vi "DAQ Initialization 4 PID.vi"(8 "error in":errorcluster, 11 "classes in":T2) -> (0 "error out":errorcluster, 3 "classes out":T2)   [LabVIEW 2011]
uses:
  Controls/Class Objects.ctl
  Modules/File/Configuration/Configuration.lvclass
  Modules/Hardware/Power Supply/Power Supply.lvclass
  Modules/Hardware/Mass Flow Controller/Mass Flow Controller.lvclass
  Modules/Hardware/PID/PID.lvclass
  Modules/Hardware/Valve Controller/Valve Controller.lvclass
  Modules/Hardware/Multimeter/Multimeter.lvclass
  Modules/Hardware/Vapour Generator/Vapour Generator.lvclass
  Modules/File/TDMS/TDMS.lvclass
  Controls/DAQ Type.ctl
  Controls/User Interface Action.ctl
  Modules/File/TDMS/File Level.ctl
  Controls/TDMS File Handling.ctl
  Functional Global Data/Device Params Global.ctl
  Functional Global Data/Run Data.ctl
  Functional Global Data/Globals.ctl
  Controls/Display Mode.ctl
  Modules/Hardware/INL PID/INL PID.lvclass
  Modules/Hardware/Baseline Mocon piD-Tech plus/Baseline Mocon piD-Tech plus.lvclass
panel:
  in  "parameter names INL PID":string[](array[string])=["Sampling Frequency", "Integration Time (ms)", "Integration Periods", "Grid Voltage", "Experiment Type", "Notes"]
  in  "Experiment Type":T1
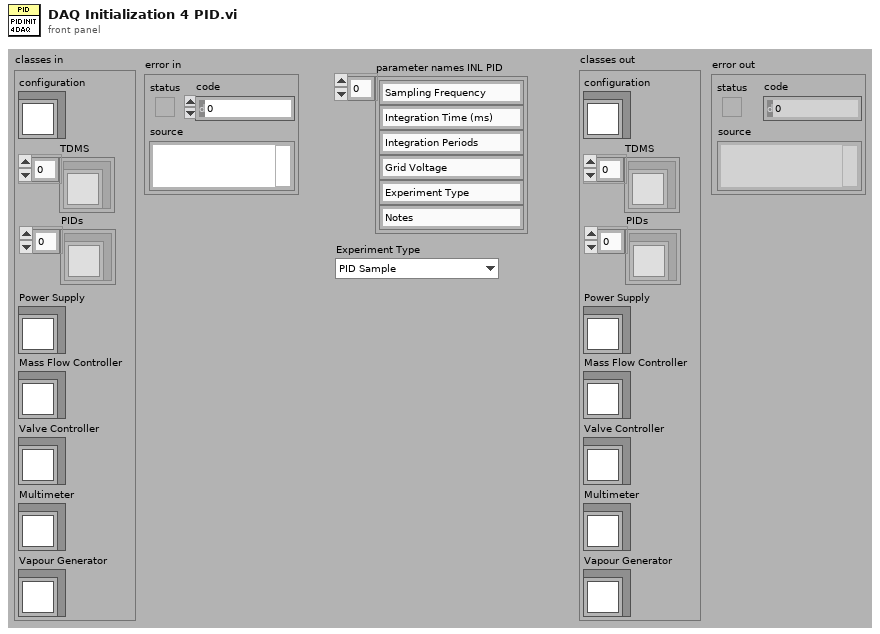
[diagram p1: front panel]
types:
  T1 = typedef "DAQ Type.ctl" = enum16{"PID Sample", "PID with PS Challenge", "PID with MFC Challenge", "Multimeter Sample", "Multimeter with MFC Challenge"}
  T2 = typedef "Class Objects.ctl" = cluster{"configuration":refnum<class "Configuration.lvclass">, "TDMS":refnum<class "TDMS.lvclass">[], "Power Supply":refnum<class "Power Supply.lvclass">, "Mass Flow Controller":refnum<class "Mass Flow Controller.lvclass">, "Valve Controller":refnum<class "Valve Controller.lvclass">, "Multimeter":refnum<class "Multimeter.lvclass">, "Vapour Generator":refnum<class "Vapour Generator.lvclass">, "PIDs":refnum<class "PID.lvclass">[]}
  T3 = typedef "User Interface Action.ctl" = enum16{"Initialize", "Data Acquisition Disable", "Data View Disable", "Sample Set", "Sample Set 2D Data", "Sample Set x0 & dx", "Sample Add", "Sample Set Cursor", "Sample Set Offset & Multiplier", "Sample Set Axis Labels", "Sample Parameters Disabled", "Sample Parameters Update", "Run Update", "Run Set Offset & Multiplier", "Run Set Axis Labels", "Run Set Cursor", "Run Set Disabled", "Run Parameters Update", "Run Parameters Disabled", "Run Number Set", "Run Number Set Range", "Run Number Set Disabled", "Sample Number Set", "Sample Number Set Range", "Notes Set Value", "Update Plot", "Set Plot Parameters", "Update Concentration Plot", "Time Set", "Clear DAQ Display", "Clear Analysis Display", "Status Bar Set", "Progress Bar Set", "Display Mode Set", "Experiment Type Set", "Analysis Plot Average Set", "Stop"}
  T4 = typedef "TDMS.lvclass/File Level.ctl" = enum16{"File", "Group", "Channel"}
  T5 = typedef "TDMS File Handling.ctl" = enum16{"Add TDMS File", "Get Active TDMS File", "Set Active TDMS File", "Set Active TDMS File Index"}
  T6 = typedef "Device Params Global.ctl" = enum16{"Initialize", "Get Device Settings", "Get Device Connections", "Set Device Settings", "Set Device Connections", "Get All Device Properties"}
  T7 = typedef "Run Data.ctl" = enum16{"Initialize", "Add Sample Channel", "Set Run", "Get Number of Runs", "Set Run Params", "Get Spectrum", "Get Run Params", "Get Sample Params", "Get History", "Get Averaged History", "Get Run Param Names", "Set Run Param Names", "Get Sample Param Names", "Set Sample Param Names", "Get MFC Flow Rate Challenge Profile", "Get History Average"}
  T8 = typedef "Globals.ctl" = enum16{"Initialize", "Get DAQ Params", "Get Data Display Params", "Set DAQ Params", "Set Data Display Params"}
  T9 = typedef "Display Mode.ctl" = enum16{"Sample", "Run"}
  T10 = typedef "Device Connections.ctl" = cluster{"Detector":cluster{"Detector Type":T11, "Connection":bool, "B-M PID":T12, "INL PID Connections":T13}, "Power Supply":cluster{"Type":enum16{"Stanford Research PS350", "Keithley 2400"}, "Connection":bool, "VISA resource name":refnum<visa-resource-name>}, "Mass Flow Controller":cluster{"Type":enum16{"Aalborg GFC17"}, "Connection":bool, "Aalborg GFC17":T15}, "Valve Controller":cluster{"Type":T16, "Connection":bool, "SMC - INL":cluster{"VISA resource name":refnum<visa-resource-name>}}, "Multimeter":cluster{"Multimeter Type":T17, "Connection":bool, "VISA resource name":refnum<visa-resource-name>}, "Vapour Generator":cluster{"Type":T18, "Connection":bool, "Owlstone Gen-SYS":T19}}
  T11 = typedef "Detector Type.ctl" = enum16{"INL PID", "Baseline-Mocon piD-TECH plus"}
  T12 = typedef "Baseline Mocon piD-Tech plus.lvclass/Connections.ctl" = cluster{"AI DAQmx channel":tag}
  T13 = typedef "INL PID Connections.ctl" = cluster{"PIDs":u8, "Integrator DAQ Channels 1":T14, "Integrator DAQ Channels 2":T14}
  T14 = typedef "INL PID.lvclass/Integrator DAQmx Channels.ctl" = cluster{"V0":tag, "S1":tag, "S2":tag}
  T15 = typedef "Aalborg GFC17.lvclass/Aalborg GFC17 Connections.ctl" = cluster{"flow rate setpoint channel":tag, "flow rate reading channel":tag, "valve channel":tag}
  T16 = typedef "Valve Type.ctl" = enum16{"SMC - INL"}
  T17 = typedef "Multimeter Type.ctl" = enum16{"Agilent 3458A"}
  T18 = typedef "Vapour Generator Type.ctl" = enum16{"Owlstone GEN-SYS"}
  T19 = typedef "Owlstone GEN-SYS.lvclass/GEN-SYS Connections.ctl" = cluster{"GEN-SYS VISA resource name":refnum<visa-resource-name>, "OVG-4":cluster{"Flow Address":u8, "Temp Address":u8}, "OHG-4":cluster{"Flow Address":u8, "Easydew VISA resource name":refnum<visa-resource-name>}}
  T20 = typedef "Device Settings.ctl" = cluster{"PID":cluster{"B-M PID":T21, "INL PID":T22}, "Power Supply":cluster{"Source Value":dbl, "Source Value Units":T23, "Source Mode":T24, "Limits":T25, "Output":bool}, "Mass Flow Controller":cluster{"MFC Flow Rate":dbl, "MFC Valve Status":T28}, "Valve Controller":cluster{"Valve Assembly":T29}, "Multimeter":cluster{"Agilent 3458A":cluster{"Measurement Configuration":T31, "Measurement Integration":T32}}, "Vapour Generator":cluster{"Owlstone Permeation Tube":T33, "Owlstone GEN-SYS Setpoints":T35}}
  T21 = typedef "Baseline Mocon piD-Tech plus.lvclass/Settings.ctl" = cluster{"Detector Sampling Frequency":dbl}
  T22 = typedef "INL PID.lvclass/Settings.ctl" = cluster{"Sampling Frequency":dbl, "Integration Time":dbl, "Integration Periods":u8, "Grid Voltage":dbl}
  T23 = typedef "Power Supply.lvclass/Source Units.ctl" = enum16{"volts", "millivolts", "microvolts", "amps", "milliamps", "microamps", "nanoamps"}
  T24 = typedef "Power Supply.lvclass/Source Mode.ctl" = enum16{"Volts", "Current"}
  T25 = typedef "Power Supply.lvclass/Protection Limits.ctl" = cluster{"Voltage Limit":dbl, "Voltage Limit Units":T26, "Current Limit":dbl, "Current Limit Units":T27, "Voltage Trip/Cmpl":dbl, "Voltage Trip/Cmpl Units":T26, "Current Trip/Cmpl":dbl, "Current Trip/Cmpl Units":T27}
  T26 = typedef "Power Supply.lvclass/Voltage Units.ctl" = enum16{"volts", "millivolts", "microvolts"}
  T27 = typedef "Power Supply.lvclass/Current Units.ctl" = enum16{"amps", "milliamps", "microamps", "nanoamps"}
  T28 = typedef "Mass Flow Controller.lvclass/Valve Status.ctl" = enum16{"Open", "Closed"}
  T29 = typedef "Valve Controller.lvclass/Valve Assembly.ctl" = cluster{"Valve 1":T30, "Valve 2":T30, "Valve 3":T30, "Valve 4":T30, "Valve 5":T30}
  T30 = typedef "Valve Controller.lvclass/Status.ctl" = u16
  T31 = typedef "Agilent 3458A.lvclass/Measurement Configuration.ctl" = cluster{"Function":enum16{"DC Voltage", "AC Voltage", "AC + DC Voltage", "DC Current", "AC Current", "AC + DC Current", "2-Wire Resistance", "4-Wire Resistance", "Frequency", "Period", "Direct Sampling DC", "Direct Sampling AC", "Sub-Sampling DC", "Sub-Sampling AC"}, " Manual Resolution":enum16{"4.5", "5.5", "6.5", "7.5", "8.5"}, "Frequency Source":enum16{"AC + DC Current", "AC + DC Voltage", "AC Current", "AC Voltage"}, "Auto Range":enum16{"OFF", "ON", "ONCE"}}
  T32 = typedef "Agilent 3458A.lvclass/Measurement Integration.ctl" = cluster{"Power Line Cycles":dbl}
  T33 = typedef "Owlstone GEN-SYS.lvclass/Permeation Tube.ctl" = cluster{"Tube":T34, "Molecular Weight":dbl, "Calibration Temperature\n(Celcius)":i32, "Permeation Rate \n(ng/min)":i32}
  T34 = typedef "Owlstone GEN-SYS.lvclass/Permeation Tube Gas.ctl" = enum16{"Isobutylene 27 Nov 2012", "Ammonia 29 Sep 2012", "DMMP Tube A 3 July 2014", "DMMP Tube B 3 July 2014"}
  T35 = typedef "Owlstone GEN-SYS.lvclass/Gen-Sys Setpoints.ctl" = cluster{"OVG-4":cluster{"Oven Temperature":i32, "Sample Flow Rate":i32, "Split Flow Status":u16, "Split Flow Rate":i32}, "OHG-4":cluster{"Wet Air Flow":i32}}
  T36 = typedef "Data Acquisition Parameters.ctl" = cluster{"Experiment Type":T1, "Experiment Name":string, "Operator Name":string, "Notes":string, "TDMS File Path":path, "Data Acquisition State":bool, "PID Voltage Sweep":T37, "MFC Challenge Profile - Heaviside Step":T38, "MFC Challenge Profile":T39, "MFC Challenge Profile - Staircase":T40}
  T37 = typedef "PID Voltage Seep Settings.ctl" = cluster{"Voltage Step (V)":dbl, "Voltage Range (V)":cluster{u16, u16}, "Time Step (s)":dbl, "Voltage Step Direction":enum16{"High 2 Low", "Low 2 High"}}
  T38 = typedef "MFC Challenge Profile - Heaviside Step.ctl" = cluster{"Valve Open Duration":u16, "MFC Flow Rate":dbl, "Valve Open Repeats":u16, "Valve Open Start":u16}
  T39 = typedef "MFC Challen Profile Type.ctl" = enum16{"Heaviside", "Staircase"}
  T40 = typedef "MFC Challenge Profile - Staircase.ctl" = cluster{"Step Time Duration":u16, "Step Flow Rate":dbl, "Steps":u16, "Valve Open Start":u16, "Recovery":bool, "Repeats":u16}
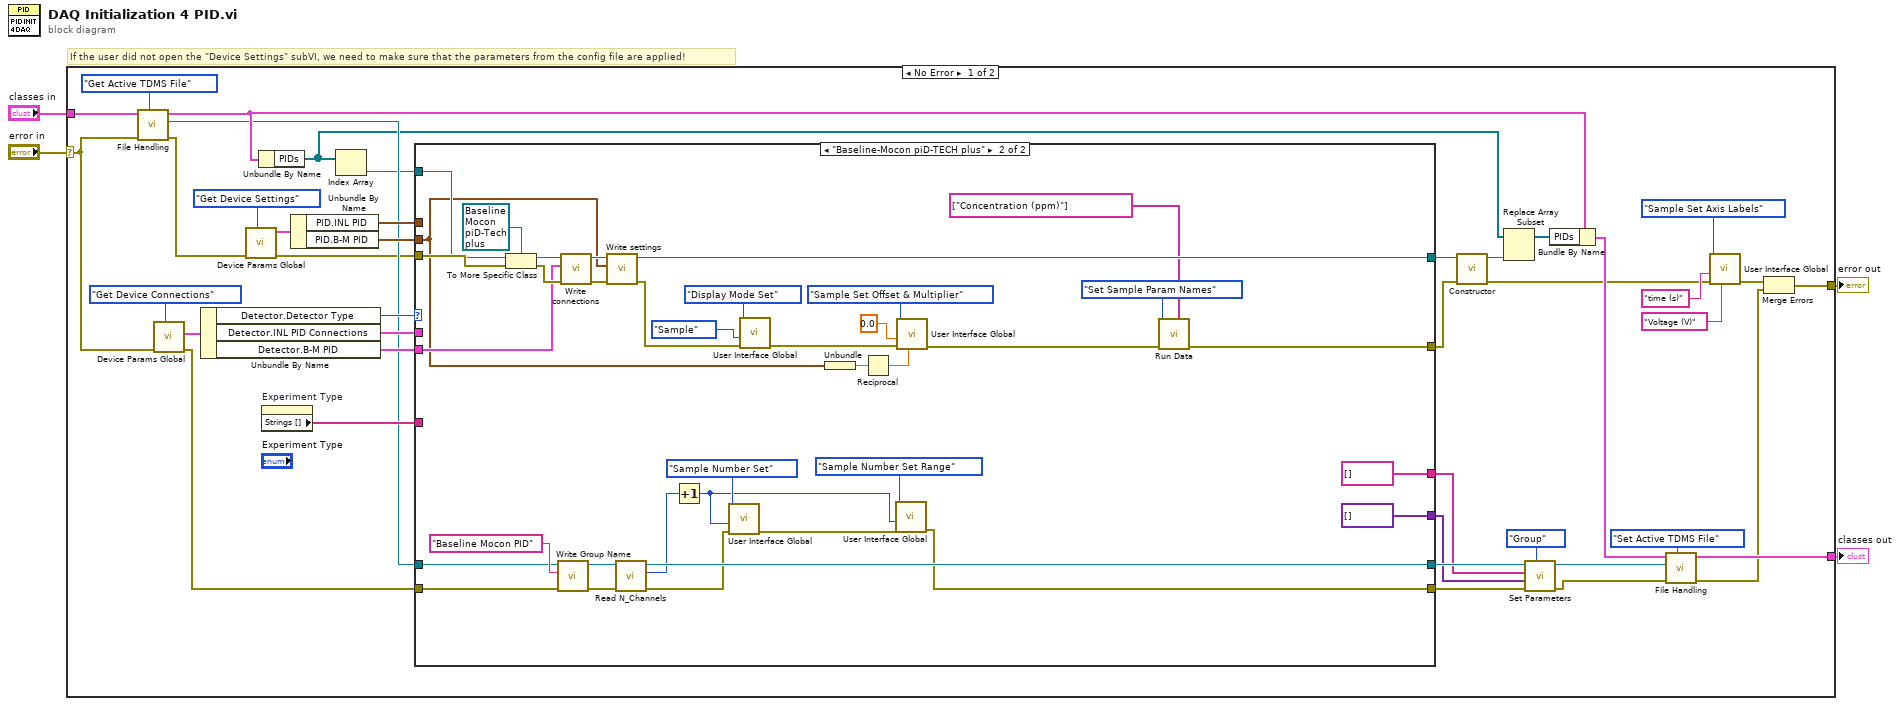
[diagram p0: block diagram]
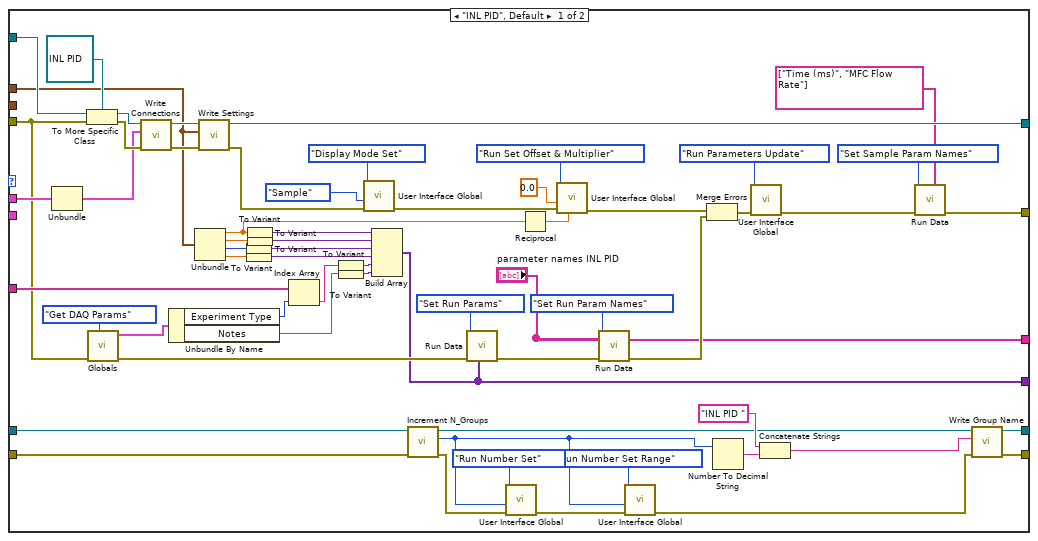
[diagram p2: hidden frame]
diagram:
  # "If the user did not open the \"Device Settings\" subVI, we need to make sure that the parameters from the config file are applied!"
  n1 = case shown="No Error" "error in" {
    selector: "error in" -> [w8 w146]
    tunnel: [w21 w146] -> w4
    tunnel: "classes in" -> [w19 w145]
    tunnel: [w36 w145] -> w1
    frame No Error {
      n2 = call "File Handling.vi"("TDMS File Handling"=TDMS_File_Handling."Get Active TDMS File", "error in"=w8, "Class objects"=w19) -> ("error out"=w6:errorcluster, "TDMS File"=w18:refnum<class "TDMS.lvclass">, "Class objects"=w20:T2)  [unwired: 6 in]
      n3 = call "Device Params Global.vi"("action"=Device_Params_Global."Get Device Connections", "error in"=w8) -> ("error out"=w7:errorcluster, "Device Connections OUT"=w42:T10)  [unwired: 7 in, 1 out]
      n4 = Unbundle By Name(w42) -> ("Detector.Detector Type"=w34:T11, "Detector.INL PID Connections"=w33:T13, "Detector.B-M PID"=w30:T12)
      n5 = call "Device Params Global.vi"("action"=Device_Params_Global."Get Device Settings", "error in"=w6) -> ("error out"=w5:errorcluster, "Device Settings OUT"=w44:T20)  [unwired: 7 in, 1 out]
      n6 = Unbundle By Name(w20) -> ("PIDs"=w11:refnum<class "PID.lvclass">[])
      n7 = property on="Experiment Type" class="Enum (strict)"() -> ("Strings []"=w27:string[])  [unwired: 2 in, 2 out]
      n8 = Unbundle By Name(w44) -> ("PID.INL PID"=w32:T22, "PID.B-M PID"=w31:T21)
      n9 = Index Array(array=w11) -> (element=w12:refnum<class "PID.lvclass">)  [unwired: 1 in]
      n10 = case shown="\"Baseline-Mocon piD-TECH plus\"" w34 {
        tunnel: w12 -> [w107 w138]
        tunnel: w5 -> [w46 w139]
        tunnel: w33 -> [w49 _]
        tunnel: w32 -> [w96 _]
        tunnel: w31 -> [_ w124]
        tunnel: [w101 w144] -> w29
        tunnel: w30 -> [_ w125]
        tunnel: w18 -> [w66 w132]
        tunnel: [w97 w116] -> w28
        tunnel: w27 -> [w85 _]
        tunnel: ["parameter names INL PID" string[] [] ("parameter names INL PID")] -> w24
        tunnel: [w72 variant[] []] -> w25
        tunnel: [w71 w108] -> w26
        tunnel: [w50 w119] -> w23
        tunnel: w7 -> [w47 w115]
        frame "INL PID", Default {
          n11 = Unbundle(w49) -> ("Integrator DAQ Channels 1"=w48:T14)  [unwired: 2 out]
          n12 = To More Specific Class(target class=refnum<class "INL PID.lvclass"> refnum ("PID.lvclass"), reference=w107, error in=w46) -> (specific class reference=w105:refnum<class "INL PID.lvclass">, error out=w104:errorcluster)
          n13 = call "Globals.vi"("action"=Globals."Get DAQ Params", "error in"=w46) -> ("error out"=w76:errorcluster, "Data Acquisition"=w87:T36)  [unwired: 7 in, 1 out]
          n14 = call-dynamic "Write Connections.vi"("error in (no error)"=w104, "Integrator DAQ Channels"=w48, "PID in"=w105) -> ("error out"=w102:errorcluster, "PID out"=w103:refnum<class "INL PID.lvclass">)  [unwired: 7 in]
          n15 = Unbundle By Name(w87) -> ("Experiment Type"=w90:T1, "Notes"=w92:string)
          n16 = Unbundle(w96) -> ("Sampling Frequency"=w54:dbl, "Integration Time"=w95:dbl, "Integration Periods"=w94:u8, "Grid Voltage"=w93:dbl)
          n17 = call-dynamic "Write Settings.vi"("error in (no error)"=w102, "INL PID"=w96, "INL PID in"=w103) -> ("error out"=w98:errorcluster, "INL PID out"=w101:refnum<class "INL PID.lvclass">)  [unwired: 7 in]
          n18 = To Variant(anything=w94) -> (Variant=w82:variant)
          n19 = To Variant(anything=w93) -> (Variant=w81:variant)
          n20 = To Variant(anything=w54) -> (Variant=w84:variant)
          n21 = To Variant(anything=w95) -> (Variant=w83:variant)
          n22 = Index Array(array=w85, index=w90) -> (element=w91:string)
          n23 = To Variant(anything=w91) -> (Variant=w86:variant)
          n24 = To Variant(anything=w92) -> (Variant=w89:variant)
          n25 = call "User Interface Global.vi"("error in"=w98, "data1"=Display_Mode."Sample" ("Display Mode"), "action"=User_Interface_Action."Display Mode Set" ("Action")) -> ("error out"=w56:errorcluster)  [unwired: 8 in]
          n26 = Build Array(w84, w83, w82, w81, w86, w89) -> (w72:variant[])
          n27 = call-dynamic "Increment N_Groups.vi"("error in"=w47, "TDMS in"=w66) -> ("error out"=w63:errorcluster, "new group number"=w62:u16, "TDMS out"=w67:refnum<class "TDMS.lvclass">)  [unwired: 7 in]
          n28 = call "Run Data.vi"("Params 1D IN"=w72, "error in"=w76, "action"=Run_Data."Set Run Params" ("Action")) -> ("error out"=w79:errorcluster)  [unwired: 5 in, 3 out]
          n29 = call "User Interface Global.vi"("error in"=w63, "data1"=w62, "action"=User_Interface_Action."Run Number Set" ("Action")) -> ("error out"=w61:errorcluster)  [unwired: 8 in]
          n30 = Reciprocal(x=w54) -> (1/x=w58:dbl)
          n31 = call "User Interface Global.vi"("data2"=w58, "error in"=w56, "data1"=0.0 ("1/x"), "action"=User_Interface_Action."Run Set Offset & Multiplier" ("Action")) -> ("error out"=w55:errorcluster)  [unwired: 7 in]
          n32 = call "Run Data.vi"("Param Names IN"="parameter names INL PID", "error in"=w79, "action"=Run_Data."Set Run Param Names" ("Action")) -> ("error out"=w75:errorcluster)  [unwired: 5 in, 3 out]
          n33 = call "User Interface Global.vi"("error in"=w61, "data1"=w62, "action"=User_Interface_Action."Run Number Set Range" ("Action")) -> ("error out"=w60:errorcluster)  [unwired: 8 in]
          n34 = Merge Errors(w55, w75) -> (w74:errorcluster)
          n35 = Number To Decimal String(number=w62) -> (decimal integer string=w69:string)  [unwired: 1 in]
          n36 = call "User Interface Global.vi"("error in"=w74, "action"=User_Interface_Action."Run Parameters Update" ("Action")) -> ("error out"=w51:errorcluster)  [unwired: 9 in]
          n37 = Concatenate Strings("INL PID " ("Group Name"), w69) -> (w68:string)
          n38 = call "Run Data.vi"("Param Names IN"=string[] ["Time (ms)", "MFC Flow Rate"], "error in"=w51, "action"=Run_Data."Set Sample Param Names" ("Action")) -> ("error out"=w50:errorcluster)  [unwired: 5 in, 3 out]
          n39 = call-dynamic "Write Group Name.vi"("error in (no error)"=w60, "Group Name"=w68, "TDMS in"=w67) -> ("error out"=w71:errorcluster, "TDMS out"=w97:refnum<class "TDMS.lvclass">)  [unwired: 7 in]
        }
        frame "Baseline-Mocon piD-TECH plus" {
          n40 = To More Specific Class(target class=refnum<class "Baseline Mocon piD-Tech plus.lvclass"> refnum ("Baseline Mocon piD-Tech plus.lvclass"), reference=w138, error in=w139) -> (specific class reference=w141:refnum<class "Baseline Mocon piD-Tech plus.lvclass">, error out=w137:errorcluster)
          n41 = call-dynamic "Write Group Name.vi"("error in (no error)"=w115, "Group Name"="Baseline Mocon PID", "TDMS in"=w132) -> ("error out"=w118:errorcluster, "TDMS out"=w117:refnum<class "TDMS.lvclass">)  [unwired: 7 in]
          n42 = call-dynamic "Write connections.vi"("error in (no error)"=w137, "Baseline-Mocon piD-TECH plus"=w125, "Baseline Mocon piD-Tech plus in"=w141) -> ("error out"=w142:errorcluster, "Baseline Mocon piD-Tech plus out"=w143:refnum<class "Baseline Mocon piD-Tech plus.lvclass">)  [unwired: 7 in]
          n43 = call-dynamic "Write settings.vi"("error in (no error)"=w142, "Baseline Mocon piD-TECH plus"=w124, "Baseline Mocon piD-Tech plus in"=w143) -> ("error out"=w135:errorcluster, "Baseline Mocon piD-Tech plus out"=w144:refnum<class "Baseline Mocon piD-Tech plus.lvclass">)  [unwired: 7 in]
          n44 = call-dynamic "Read N_Channels.vi"("error in"=w118, "TDMS.lvclass in"=w117) -> ("error out"=w112:errorcluster, "N_Channels"=w114:u16, "TDMS.lvclass out"=w116:refnum<class "TDMS.lvclass">)  [unwired: 7 in]
          n45 = Increment(x=w114) -> (x+1=w110:u16)
          n46 = call "User Interface Global.vi"("error in"=w112, "data1"=w110, "action"=User_Interface_Action."Sample Number Set" ("Action")) -> ("error out"=w109:errorcluster)  [unwired: 8 in]
          n47 = call "User Interface Global.vi"("error in"=w135, "data1"=Display_Mode."Sample" ("Display Mode"), "action"=User_Interface_Action."Display Mode Set" ("Action")) -> ("error out"=w126:errorcluster)  [unwired: 8 in]
          n48 = Unbundle(w124) -> ("Detector Sampling Frequency"=w123:dbl)
          n49 = Reciprocal(x=w123) -> (1/x=w128:dbl)
          n50 = call "User Interface Global.vi"("error in"=w109, "data1"=w110, "action"=User_Interface_Action."Sample Number Set Range" ("Action")) -> ("error out"=w108:errorcluster)  [unwired: 8 in]
          n51 = call "User Interface Global.vi"("data2"=w128, "error in"=w126, "data1"=0.0 ("1/x"), "action"=User_Interface_Action."Sample Set Offset & Multiplier" ("Action")) -> ("error out"=w120:errorcluster)  [unwired: 7 in]
          n52 = call "Run Data.vi"("Param Names IN"=string[] ["Concentration (ppm)"], "error in"=w120, "action"=Run_Data."Set Sample Param Names" ("Action")) -> ("error out"=w119:errorcluster)  [unwired: 5 in, 3 out]
        }
      }
      n53 = call-dynamic "Constructor.vi"("error in"=w23, "Detector in"=w29) -> ("error out"=w15:errorcluster, "Detector out"=w10:refnum<class "PID.lvclass">)  [unwired: 7 in, 1 out]
      n54 = Replace Array Subset(array=w11, new element=w10) -> (w9:refnum<class "PID.lvclass">[])  [unwired: 1 in]
      n55 = call-dynamic "Set Parameters.vi"("File Level"=File_Level."Group", "error in (no error)"=w26, "property values"=w25, "property names"=w24, "TDMS.lvclass in"=w28) -> ("error out"=w35:errorcluster, "TDMS.lvclass out"=w37:refnum<class "TDMS.lvclass">)  [unwired: 5 in]
      n56 = Bundle By Name(cluster=w20, "PIDs"=w9) -> (w40:T2)
      n57 = call "File Handling.vi"("TDMS File Handling"=TDMS_File_Handling."Set Active TDMS File", "error in"=w35, "TDMS File"=w37, "Class objects"=w40) -> ("error out"=w22:errorcluster, "Class objects"=w36:T2)  [unwired: 5 in, 1 out]
      n58 = call "User Interface Global.vi"("data2"="Voltage (V)", "error in"=w15, "data1"="time (s)", "action"=User_Interface_Action."Sample Set Axis Labels") -> ("error out"=w14:errorcluster)  [unwired: 7 in]
      n59 = Merge Errors(w14, w22) -> (w21:errorcluster)
    }
    frame Error {
    }
  }
  "error out" <- w4
  "classes out" <- w1
